vi "CleanUp Shell.vi"(8 "error in (no error)":errorcluster) -> (0 "error out":errorcluster)   [LabVIEW 2019, in "LabVIEW-ProviderShell.lvlib" / "LvProviderShellHelper.lvclass"]
uses:
  LvProviderShellHelper.lvclass
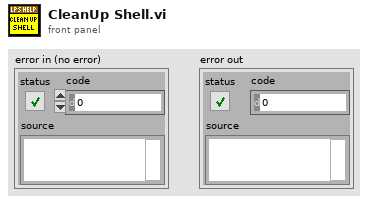
[diagram p1: front panel]
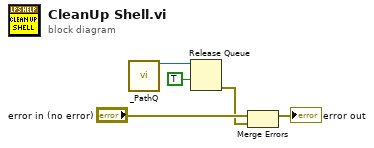
[diagram p0: block diagram]
diagram:
  n1 = call "_PathQ.vi"() -> ("Queue out"=w4:refnum<queue>)  [unwired: 10 in, 1 out]
  n2 = Release Queue(queue=w4, force destroy? (F)=TRUE) -> (error out=w1:errorcluster)  [unwired: 1 in, 2 out]
  n3 = Merge Errors("error in (no error)", w1) -> (→"error out":errorcluster)
